vi "absolute_orientation.vi"(7 "doScale":bool=TRUE, 8 "error in":errorcluster, 9 "Mapped To":dbl[][](array[numeric])=[[0.0, -1.0, -1.0], [1.0, 1.0, 0.0]], 11 "Mapped From":dbl[][](array[numeric])=[[3.0, 3.0, 1.0], [1.0, 3.0, 3.0]]) -> (0 "error out":errorcluster, 1 "least squares error":dbl, 3 "transformation_description":dbl[](array[numeric]))   [LabVIEW 2019]
uses:
  <vilib>/imath/engines/lvmath2/RunTimeEngine/BuiltInFunctions/mean/NIMS_RCol=mean(RM,I32).vi
  <vilib>/imath/engines/lvmath2/RunTimeEngine/BuiltInFunctions/size/NIMS_I32=size(GM,I32).vi
  <instcachedir>/0/NIMS_I32=size(GM,I32)_68C934A652CA42C4B4FC52616FF9B860.lvgen/NIMS_I32=size(GM,I32)_68C934A652CA42C4B4FC52616FF9B860_004.vi
  <vilib>/imathl/engines/lvmath/Functions/Error Handling/Create Error.vi
  <vilib>/imath/engines/lvmath2/RunTimeEngine/RangeToken/NIMS_Range_R2 - Integer.vi
  <instcachedir>/0/NIMS_Range_R2 - Integer_5118B3908D7D4A9BA0DEB8EE73549D2D.lvgen/NIMS_Range_R2 - Integer_5118B3908D7D4A9BA0DEB8EE73549D2D_000.vi
  <vilib>/imath/engines/lvmath2/RunTimeEngine/CommandStatement/MC_CommandStatement_break.vi
  <vilib>/imath/engines/lvmath2/RunTimeEngine/IndexRead/NIMS M(S,$).vi
  <instcachedir>/0/NIMS M(S,$)_F24F360562DE41D8BE234322A2E15C65.lvgen/NIMS M(S,$)_F24F360562DE41D8BE234322A2E15C65_000.vi
  <vilib>/imath/engines/lvmath2/RunTimeEngine/IndexRead/NIMS V(S).vi
  <instcachedir>/0/NIMS V(S)_0488751826AF41519A22953C041130DC.lvgen/NIMS V(S)_0488751826AF41519A22953C041130DC_000.vi
  <vilib>/imath/engines/lvmath2/RunTimeEngine/IndexReplace/NIMS M(S,$)=V.vi
  <instcachedir>/0/NIMS M(S,$)=V_A09479BBA4444DECA290951A14C35476.lvgen/NIMS M(S,$)=V_A09479BBA4444DECA290951A14C35476_000.vi
  <vilib>/imath/engines/lvmath2/RunTimeEngine/ErrorHandling/NIMS_Create Error From Enums.vi
  <vilib>/imath/engines/lvmath2/RunTimeEngine/ArithmeticOperatorToken/NIMS_ArithmeticOperator_multmx.vi
  <instcachedir>/0/NIMS_ArithmeticOperator_multmx_99144D996F2B45CCBE745A128A95DE55.lvgen/NIMS_ArithmeticOperator_multmx_99144D996F2B45CCBE745A128A95DE55_004.vi
  <vilib>/imath/engines/lvmath2/RunTimeEngine/IndexRead/NIMS M(S).vi
  <instcachedir>/0/NIMS M(S)_B826C018497E4940AE96BD27B540B6FB.lvgen/NIMS M(S)_B826C018497E4940AE96BD27B540B6FB_000.vi
  <vilib>/imath/engines/lvmath2/RunTimeEngine/BuiltInFunctions/eig/NIMS_[CM,CM]=eig(M).vi
  <instcachedir>/0/NIMS_[CM,CM]=eig(M)_D108A2703E184A34AECDE3AAB68F928B.lvgen/NIMS_[CM,CM]=eig(M)_D108A2703E184A34AECDE3AAB68F928B_000.vi
  <vilib>/imath/engines/lvmath2/RunTimeEngine/ErrorHandling/NIMS_Error From Error Code.vi
  <vilib>/imath/engines/lvmath2/RunTimeEngine/BuiltInFunctions/diag/NIMS_diag.vi
  <instcachedir>/0/NIMS_diag_6FE20E45AD3542C1A51E40EF10B25DE1.lvgen/NIMS_diag_6FE20E45AD3542C1A51E40EF10B25DE1_002.vi
  <vilib>/imath/engines/lvmath2/RunTimeEngine/BuiltInFunctions/max/1 input/NIMS_max(RM).vi
  <instcachedir>/0/NIMS_max(RM)_2A49E9E607A849919E26F1E5E1595B35.lvgen/NIMS_max(RM)_2A49E9E607A849919E26F1E5E1595B35_000.vi
  <instcachedir>/0/NIMS V(S)_0488751826AF41519A22953C041130DC.lvgen/NIMS V(S)_0488751826AF41519A22953C041130DC_002.vi
  <vilib>/imath/engines/lvmath2/RunTimeEngine/IndexRead/NIMS M($,S).vi
  <instcachedir>/0/NIMS M($,S)_3E5749BBB62E49528D4765A77F1F6D98.lvgen/NIMS M($,S)_3E5749BBB62E49528D4765A77F1F6D98_001.vi
  <vilib>/imath/engines/lvmath2/RunTimeEngine/BuiltInFunctions/norm/NIMS_norm(GV,DBL).vi
  <instcachedir>/0/NIMS_norm(GV,DBL)_1701EDF462C84E9CAEC5A1EAB8C3AC13.lvgen/NIMS_norm(GV,DBL)_1701EDF462C84E9CAEC5A1EAB8C3AC13_000.vi
  <vilib>/imath/engines/lvmath2/RunTimeEngine/BuiltInFunctions/prod/NIMS_prod(GV).vi
  <instcachedir>/0/NIMS_prod(GV)_1D7C69903E9744BFBC8310E18FF565A3.lvgen/NIMS_prod(GV)_1D7C69903E9744BFBC8310E18FF565A3_000.vi
  <vilib>/imath/engines/lvmath2/RunTimeEngine/ArithmeticOperatorToken/NIMS_ArithmeticOperator_multmx(M,CV).vi
  <instcachedir>/0/NIMS_ArithmeticOperator_multmx(M,CV)_189E65F7C3284A1CB75AED062D0FBD41.lvgen/NIMS_ArithmeticOperator_multmx(M,CV)_189E65F7C3284A1CB75AED062D0FBD41_000.vi
  <vilib>/imath/engines/lvmath2/RunTimeEngine/ArithmeticOperatorToken/NIMS_ArithmeticOperator_minus.vi
  <instcachedir>/0/NIMS_ArithmeticOperator_minus_A2D45F688BFF4915B286240799BA2370.lvgen/NIMS_ArithmeticOperator_minus_A2D45F688BFF4915B286240799BA2370_002.vi
  <vilib>/imath/engines/lvmath2/RunTimeEngine/ArithmeticOperatorToken/NIMS_ArithmeticOperator_times.vi
  <instcachedir>/0/NIMS_ArithmeticOperator_times_BC2A7BF92F8245379E8C6B3F6BDCD4B7.lvgen/NIMS_ArithmeticOperator_times_BC2A7BF92F8245379E8C6B3F6BDCD4B7_007.vi
  <vilib>/imath/engines/lvmath2/RunTimeEngine/IndexRead/NIMS M($).vi
  <instcachedir>/0/NIMS M($)_82D1177398184AFB96A6AFB63C3C3F57.lvgen/NIMS M($)_82D1177398184AFB96A6AFB63C3C3F57_000.vi
  <vilib>/imath/engines/lvmath2/RunTimeEngine/BuiltInFunctions/sum/NIMS_sum(GV).vi
  <instcachedir>/0/NIMS_sum(GV)_67F5EC36BC034E54A6BEC5B0673C00E5.lvgen/NIMS_sum(GV)_67F5EC36BC034E54A6BEC5B0673C00E5_000.vi
  <vilib>/imath/engines/lvmath2/RunTimeEngine/BuiltInFunctions/atan2/NIMS_atan2.vi
  <instcachedir>/0/NIMS_atan2_A91AA4A7D42247EDBE8F76DB99AF04A4.lvgen/NIMS_atan2_A91AA4A7D42247EDBE8F76DB99AF04A4_000.vi
  <vilib>/imath/engines/lvmath2/RunTimeEngine/NodeEndStatement/NIMS_NodeEndStatement_Output.vi
  <instcachedir>/0/NIMS_NodeEndStatement_Output_53EC0D466D134D7ABD903AC30B43404B.lvgen/NIMS_NodeEndStatement_Output_53EC0D466D134D7ABD903AC30B43404B_005.vi
  <vilib>/imath/engines/lvmath2/RunTimeEngine/ErrorHandling/NIMS_Finalize Error.vi
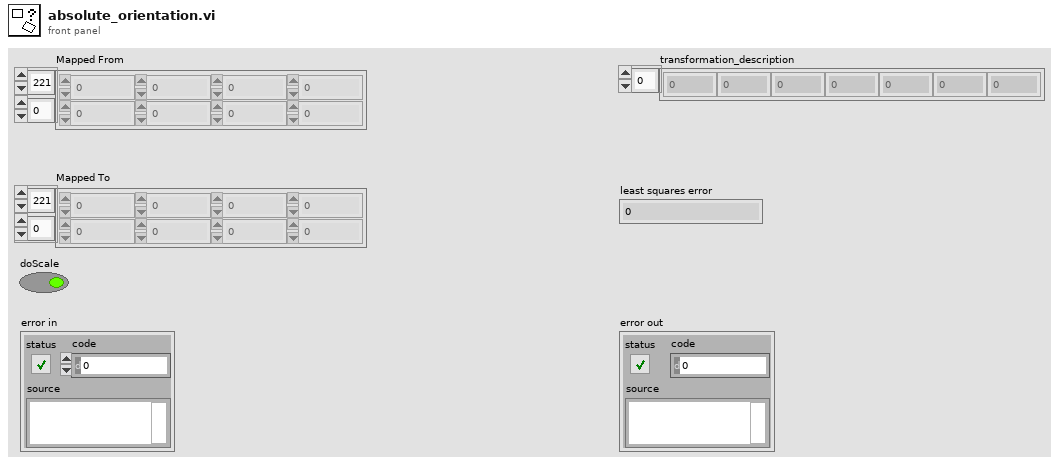
[diagram p1: front panel]
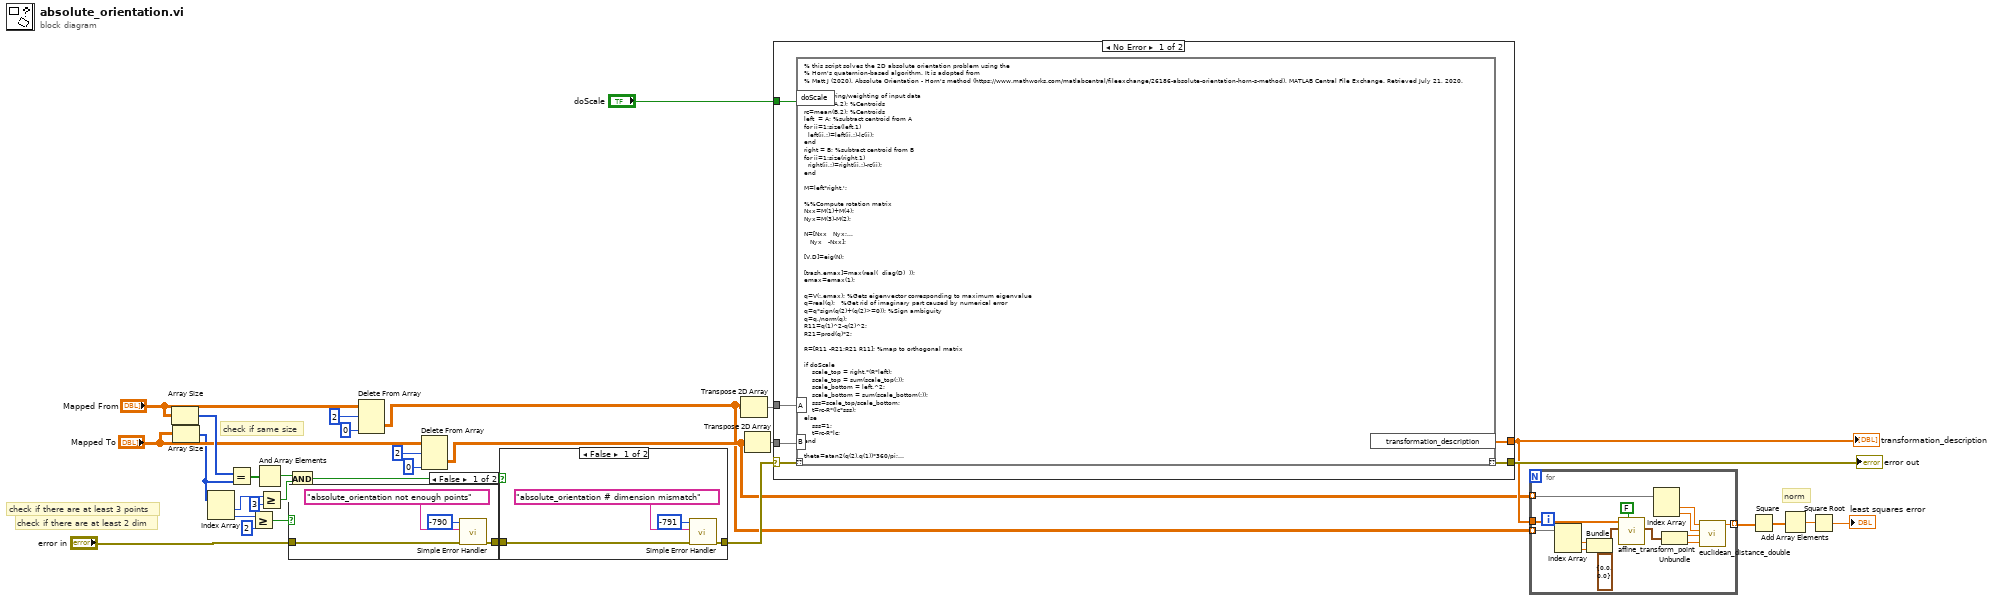
[diagram p0: block diagram]
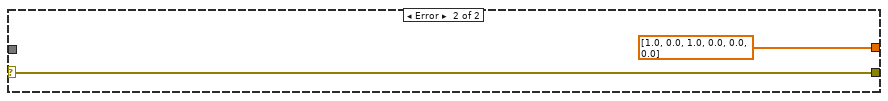
[diagram p4: hidden frame]
diagram:
  # "check if there are at least 2 dim"
  # "check if there are at least 3 points"
  # "check if same size"
  # "norm"
  n1 = Array Size(array="Mapped From") -> (size(s)=w26:i32[])
  n2 = Array Size(array="Mapped To") -> (size(s)=w7:i32[])
  n3 = Index Array(array=w7) -> (element #1=w6:i32, element #2=w5:i32)  [unwired: 2 in]
  n4 = Equal?(x=w26, y=w7) -> (x = y?=w25:bool[])
  n5 = Greater Or Equal?(x=w5, y=2) -> (x >= y?=w21:bool)
  n6 = And Array Elements(Boolean array=w25) -> (logical AND=w20:bool)
  n7 = Greater Or Equal?(x=w6, y=3) -> (x >= y?=w19:bool)
  n8 = case shown="False" w21 {
    tunnel: "error in" -> [w35 w36]
    tunnel: [w34 w36] -> w18
    frame False {
      n9 = call <vilib>:"Simple Error Handler.vi"("error code (no error:0)"=-790, "error source (\" \")"="absolute_orientation not enough points" ("error source (\" \")"), "error in (no error)"=w35) -> ("error out"=w34:errorcluster)  [unwired: 2 in, 4 out]
    }
    frame True {
    }
  }
  n10 = And(x=w20, y=w19) -> (x .and. y?=w16:bool)
  n11 = Delete From Array(array="Mapped From", length=2, index (col)=0 ("disabled index (col)")) -> (deleted portion=w1:dbl[][])  [unwired: 1 in, 1 out]
  n12 = Delete From Array(array="Mapped To", length=2, index (col)=0 ("disabled index (col)")) -> (deleted portion=w2:dbl[][])  [unwired: 1 in, 1 out]
  n13 = case shown="False" w16 {
    tunnel: w18 -> [w40 w41]
    tunnel: [w39 w41] -> w17
    frame False {
      n14 = call <vilib>:"Simple Error Handler.vi"("error code (no error:0)"=-791, "error source (\" \")"="absolute_orientation # dimension mismatch" ("error source (\" \")"), "error in (no error)"=w40) -> ("error out"=w39:errorcluster)  [unwired: 2 in, 4 out]
    }
    frame True {
    }
  }
  n15 = Transpose 2D Array(2D array=w1) -> (transposed array=w4:dbl[][])
  n16 = Transpose 2D Array(2D array=w2) -> (transposed array=w3:dbl[][])
  n17 = case shown="No Error" w17 {
    selector: w17 -> [w42 w726]
    tunnel: "doScale" -> [w47 _]
    tunnel: [w46 dbl[] [1.0, 0.0, 1.0, 0.0, 0.0, 0.0] ("transformation_description")] -> w15
    tunnel: w4 -> [w45 _]
    tunnel: w3 -> [w44 _]
    tunnel: [w43 w726] -> w23
    frame No Error {
      n18 = mathscript code="% this script solves the 2D absolute orientation problem using the\n% Horn's quaternion-based algorithm. It is adopted from \n% Matt J (2020). Absolute Orientation - Horn's method (https://www.mathworks.com/matlabcentral/fileexchange/26186-absolute-orientation-horn-s-method), MATLAB Central File Exchange. Retrieved July 21, 2020.\n\n%%Centering/weighting of input data\nlc=mean(A,2); %Centroids\nrc=mean(B,2); %Centroids\nleft  = A; %subtract centroid from A\nfor ii=1:size(left,1)\n  left(ii,:)=left(ii,:)-lc(ii);\nend\nright = B; %subtract centroid from B\nfor ii=1:size(right,1)\n  right(ii,:)=right(ii,:)-rc(ii);\nend\n \nM=left*right.';\n\n%%Compute rotation matrix\nNxx=M(1)+M(4); \nNyx=M(3)-M(2);\n\nN=[Nxx   Nyx;...\n   Nyx   -Nxx];\n\n[V,D]=eig(N);\n\n[trash,emax]=max(real(  diag(D)  ));\nemax=emax(1);\n\nq=V(:,emax); %Gets eigenvector corresponding to maximum eigenvalue\nq=real(q);   %Get rid of imaginary part caused by numerical error\nq=q*sign(q(2)+(q(2)>=0)); %Sign ambiguity\nq=q./norm(q);\nR11=q(1)^2-q(2)^2;\nR21=prod(q)*2;\n\nR=[R11 -R21;R21 R11]; %map to orthogonal matrix\n\nif doScale\n    scale_top = right.*(R*left);\n    scale_top = sum(scale_top(:));\n    scale_bottom = left.^2;\n    scale_bottom = sum(scale_bottom(:));\n    sss=scale_top/scale_bottom;\n    t=rc-R*(lc*sss);\nelse\n    sss=1;\n    t=rc-R*lc;\nend\n\ntheta=atan2(q(2),q(1))*360/pi;\ntransformation_description = [R11, R21, sss, t(1), t(2), theta];\n%Bfit=(sss*R)*A;\n%%apply translation\n%for ii=1:size(Bfit,1)\n%  Bfit(ii,:)=Bfit(ii,:)+t(ii);\n%end\n\n%BfmB = Bfit-B;\n%err=sqrt(sum(BfmB.^2,1)); %l2 norm\n%errlsq=norm(err); %unnormalize the weights\n%errmax=max(err);"("??"=w42, "A"=w45, "B"=w44, "doScale"=w47) -> ("??"=w43:errorcluster, "transformation_description"=w46:dbl[])
    }
    frame Error {
    }
  }
  "transformation_description" <- w15
  "error out" <- w23
  n19 = for {
    tunnel: [w741] -> w30 mode=indexing
    tunnel: w2 -> [w740] mode=indexing
    tunnel: w15 -> [w737]
    tunnel: w1 -> [w736] mode=indexing
    n20 = Index Array(array=w736) -> (element #1=w735:dbl, element #2=w734:dbl)  [unwired: 2 in]
    n21 = Bundle(cluster=cluster{"X":sgl, "Y":sgl} {"X"=0.0, "Y"=0.0} ("Pixel Coordinates In"), "X"=w735, "Y"=w734) -> (w732:cluster{"X":sgl, "Y":sgl})
    n22 = call "affine_transform_point.vi"("Inverse Transform"=FALSE, "Pixel Coordinates In"=w732, "transformation_description"=w737) -> ("Pixel Coordinates Out"=w731:cluster{"X":sgl, "Y":sgl})  [unwired: 8 in]
    n23 = Index Array(array=w740) -> (element #1=w739:dbl, element #2=w738:dbl)  [unwired: 2 in]
    n24 = Unbundle(w731) -> ("X"=w730:sgl, "Y"=w729:sgl)
    n25 = call "euclidean_distance_double.vi"("Point 2 Y"=w729, "Point 2 X"=w730, "Point 1 Y"=w738, "Point 1 X"=w739) -> ("Distance"=w741:dbl)  [unwired: 7 in]
  }
  n26 = Square(x=w30) -> (x^2=w29:dbl[])
  n27 = Add Array Elements(numeric array=w29) -> (sum=w28:dbl)
  n28 = Square Root(x=w28) -> (sqrt(x)=→"least squares error":dbl)
